vi "Queue Release.vi"(8 "error in (no error)":errorcluster caption="Error In", 11 "Queue In":refnum<queue>) -> (0 "error out":errorcluster caption="Error Out")   [LabVIEW 2020]
uses:
  Queue Message.ctl
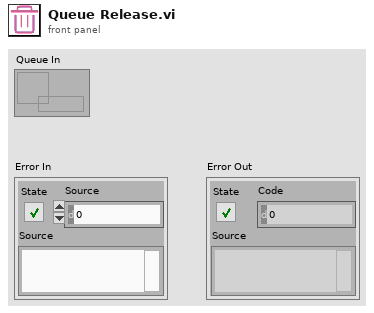
[diagram p1: front panel]
types:
  T1 = enum16{"Read Queue", "Add Queue", "Delete Queue"}
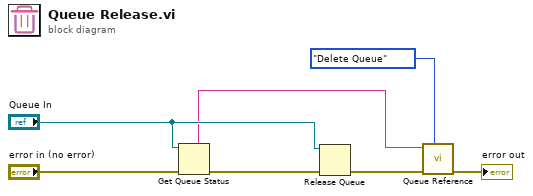
[diagram p0: block diagram]
diagram:
  n1 = Get Queue Status(queue="Queue In", error in (no error)="error in (no error)") -> (queue name=w3:string, error out=w5:errorcluster)  [unwired: 1 in, 6 out]
  n2 = Release Queue(queue="Queue In", error in (no error)=w5) -> (error out=w2:errorcluster)  [unwired: 1 in, 2 out]
  n3 = call "Queue Reference.vi"("Mode"=T1."Delete Queue", "Error In"=w2, "Name"=w3) -> ("Error Out"=→"error out":errorcluster)  [unwired: 5 in, 3 out]
